vi "Data Destroy.vi"(8 "error in (no error)":errorcluster, 11 "Data DVR in":refnum<data-value>) -> (0 "error out":errorcluster)   [LabVIEW 2012, in "MDSplus.lvlib"]
uses:
  <vilib>/MDSplus/Library/MDSplus.lvlib
  <vilib>/MDSplus/Classes/Data_Class/Data.lvclass
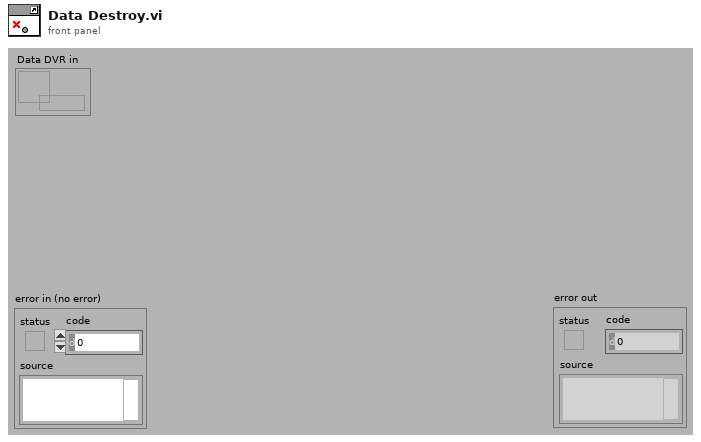
[diagram p1: front panel]
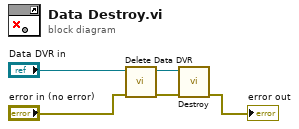
[diagram p0: block diagram]
diagram:
  n1 = call <vilib>:"Delete Data DVR.vi"("error in (no error)"="error in (no error)", "Data DVR in"="Data DVR in") -> ("error out"=w2:errorcluster, "Data out"=w3:refnum<class "Data.lvclass">)  [unwired: 8 in]
  n2 = call-dynamic "Destroy.vi"("error in (no error)"=w2, "Data in"=w3) -> ("error out"=→"error out":errorcluster)  [unwired: 9 in]
